vi "Mod_OFDM_Remove_Cyclic_Prefix_Frame.vi"(0 "output complex\nwaveform":T1 {"Y" format="%.3f"; "dt" format="%^.2e"; "t0" format="%.4f"}, 5 "Offset":i32, 11 "error in (no error)":errorcluster, 13 "Parameters per Ofdm Symbol":T2 {"Data Source"."Data Source"."Register Initial State" format="%08x"}) -> (2 "FFT o/p":cdb[](array[numeric]), 4 "FFT {X}":cdb[][](array[numeric]), 15 "error out":errorcluster)   [LabVIEW 2010]
uses:
  Controls(Type_DEf)/Parameters per Ofdm Symbol.ctl
  <vilib>/addons/Modulation/Analog/controls/Complex Data Waveform.ctl
  <vilib>/Analysis/2dsp.llb/Complex FFT.vi
  <vilib>/Analysis/NI_AALPro.lvlib
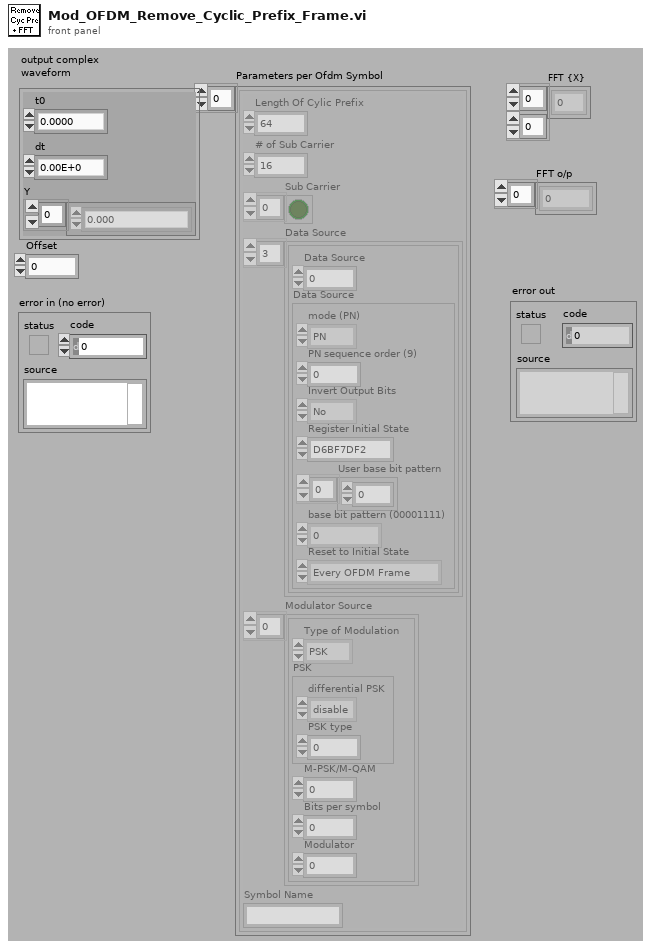
[diagram p1: front panel]
types:
  T1 = typedef "Complex Data Waveform.ctl" = cluster{"t0":dbl, "dt":dbl, "Y":cdb[]}
  T2 = typedef "Parameters per Ofdm Symbol.ctl" = cluster{"Length Of Cylic Prefix":i32, "# of Sub Carrier":i32, "Sub Carrier":bool[], "Data Source":cluster{"Data Source":u16, "Data Source":cluster{"mode (PN)":enum16{"PN", "pattern", "user"}, "PN sequence order (9)":i32, "Invert Output Bits":enum16{"No", "Yes"}, "Register Initial State":u32, "User base bit pattern":i8[], "base bit pattern (00001111)":enum16{"0", "1", "01", "0011", "00001111"}, "Reset to Initial State":enum16{"Every OFDM Frame", "Every OFDM Symbol", "Every Sub Carrier"}}}[], "Modulator Source":cluster{"Type of Modulation":enum16{"PSK", "QAM"}, "PSK":cluster{"differential PSK":enum16{"disable", "enable"}, "PSK type":u16}, "M-PSK/M-QAM":i32, "Bits per symbol":i32, "Modulator":u16}[], "Symbol Name":string}[]
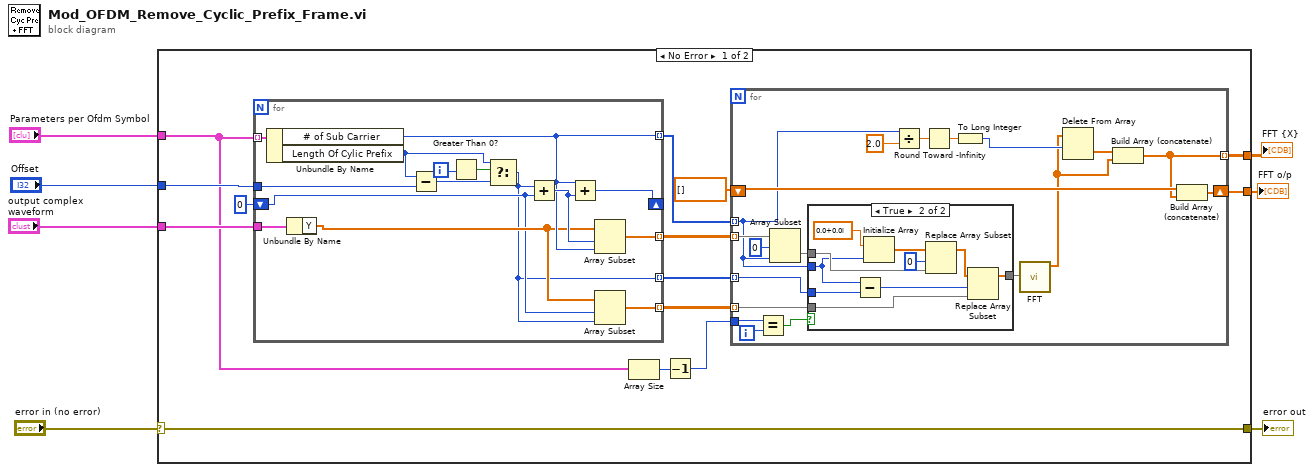
[diagram p0: block diagram]
diagram:
  n1 = case shown="No Error" "error in (no error)" {
    selector: "error in (no error)" -> [w9 w67]
    tunnel: "output complex\nwaveform" -> [w21 _]
    tunnel: "Offset" -> [w20 _]
    tunnel: "Parameters per Ofdm Symbol" -> [w15 _]
    tunnel: [w10 _] -> w4
    tunnel: [w9 w67] -> w2
    tunnel: [w8 _] -> w1
    frame No Error {
      n2 = for {
        tunnel: w15 -> [w65] mode=indexing
        tunnel: w21 -> [w66]
        tunnel: w20 -> [w62]
        shift-right: [w59] -> _
        shift-left: 0 -> [w55]
        tunnel: [w58] -> w17 mode=indexing
        tunnel: [w57] -> w18 mode=indexing
        tunnel: [w54] -> w12 mode=indexing
        tunnel: [w52] -> w16 mode=indexing
        i -> [w64]
        n3 = Unbundle By Name(w65) -> ("# of Sub Carrier"=w57:i32, "Length Of Cylic Prefix"=w53:i32)
        n4 = Unbundle By Name(w66) -> ("Y"=w56:cdb[])
        n5 = Subtract(x=w53, y=w62) -> (x-y=w61:i32)
        n6 = Greater Than 0?(x=w64) -> (x > 0?=w63:bool)
        n7 = Select(t=w53, s=w63, f=w61) -> (s? t:f=w52:i32)
        n8 = Add(x=w52, y=w55) -> (x+y=w60:i32)
        n9 = Add(x=w57, y=w60) -> (x+y=w59:i32)
        n10 = Array Subset(array=w56, index=w60, length=w57) -> (w58:cdb[])
        n11 = Array Subset(array=w56, index=w55, length=w52) -> (w54:cdb[])
      }
      n12 = Array Size(array=w15) -> (size(s)=w14:i32)
      n13 = Decrement(x=w14) -> (x-1=w13:i32)
      n14 = for {
        tunnel: w17 -> [w39] mode=indexing
        tunnel: w18 -> [w29] mode=indexing
        tunnel: w12 -> [w34] mode=indexing
        tunnel: w16 -> [w33] mode=indexing
        tunnel: w13 -> [w37]
        shift-right: [w31] -> w10
        shift-left: cdb[] [] -> [w30]
        tunnel: [w22] -> w8 mode=indexing
        i -> [w38]
        n15 = Equal?(x=w37, y=w38) -> (x = y?=w36:bool)
        n16 = Array Subset(array=w39, index=0, length=w29) -> (w35:cdb[])
        n17 = case shown="True" w36 {
          tunnel: w29 -> [_ w45]
          tunnel: w35 -> [w41 w48]
          tunnel: w34 -> [_ w46]
          tunnel: w33 -> [_ w44]
          tunnel: [w41 w42] -> w32
          frame False {
          }
          frame True {
            n18 = Subtract(x=w45, y=w44) -> (x-y=w43:i32)
            n19 = Initialize Array(cdb 0.0+0.0i, w45) -> (w50:cdb[])
            n20 = Replace Array Subset(array=w50, new element=w48, index=0) -> (w47:cdb[])
            n21 = Replace Array Subset(array=w47, new element=w46, index=w43) -> (w42:cdb[])
          }
        }
        n22 = Divide(x=w29, y=2.0) -> (x/y=w27:dbl)
        n23 = Round Toward -Infinity(1:w27) -> (0:w26:dbl)
        n24 = To Long Integer(number=w26) -> (32bit integer=w25:i32)
        n25 = call-poly <vilib>:"FFT.vi"("X"=w32) -> ("FFT {X}"=w23:cdb[])  [unwired: 9 in, 1 out]
        n26 = Delete From Array(array=w23, length=w25) -> (deleted portion=w24:cdb[])  [unwired: 1 in, 1 out]
        n27 = Build Array (concatenate)(w24, w23) -> (w22:cdb[])
        n28 = Build Array (concatenate)(w30, w22) -> (w31:cdb[])
      }
    }
    frame Error {
    }
  }
  "FFT {X}" <- w1
  "error out" <- w2
  "FFT o/p" <- w4
